vi "Launch Smart Relay Actor.vi"(8 "error in":errorcluster, 11 "SCADA in":refnum<class "EMS.lvclass">) -> (0 "error out":errorcluster, 3 "SCADA out":refnum<class "EMS.lvclass">)   [LabVIEW 2018, in "EMS Core.lvlib" / "EMS.lvclass"]
uses:
  EMS.lvclass
  C:/Users/Administrator/Desktop/LabVIEW EMS/EMS Generic Actor/EMS Generic/EMS Generic.lvclass
  C:/Program Files (x86)/National Instruments/LabVIEW 2018/vi.lib/ActorFramework/Actor/Actor.lvclass
  IED Actors/Smart Relay Actor/Smart Relay/Smart Relay.lvclass
  <vilib>/ORNL/CSEISMIC DDS/CSEISMIC DDS Base/Data Types/Controls/DeviceClass Selector.ctl
  EMS.lvclass/EMS.ctl
  <vilib>/ActorFramework/Actor/Actor.lvclass
  <vilib>/ORNL/CSEISMIC DDS/CSEISMIC DDS Base/CSEISMIC DDS.lvclass
  EMS Generic Actor/EMS Generic/EMS Generic.lvclass
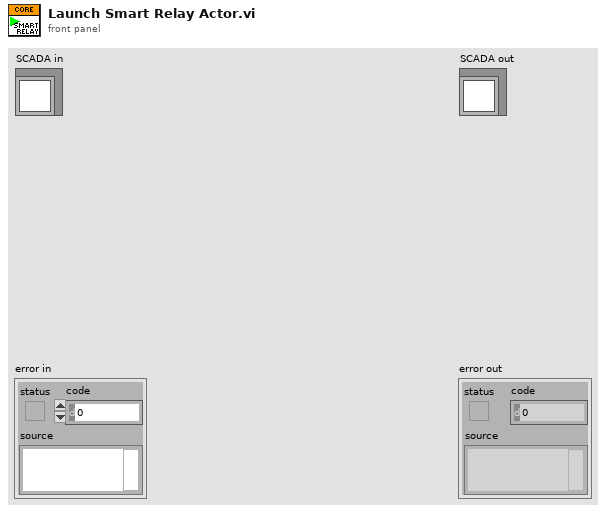
[diagram p1: front panel]
types:
  T1 = typedef "CSEISMIC DDS.lvlib/CSEISMIC DDS.lvclass/DeviceID.ctl" = string
  T2 = typedef "CSEISMIC DDS.lvlib/CSEISMIC DDS.lvclass/DeviceClass Selector.ctl" = u16
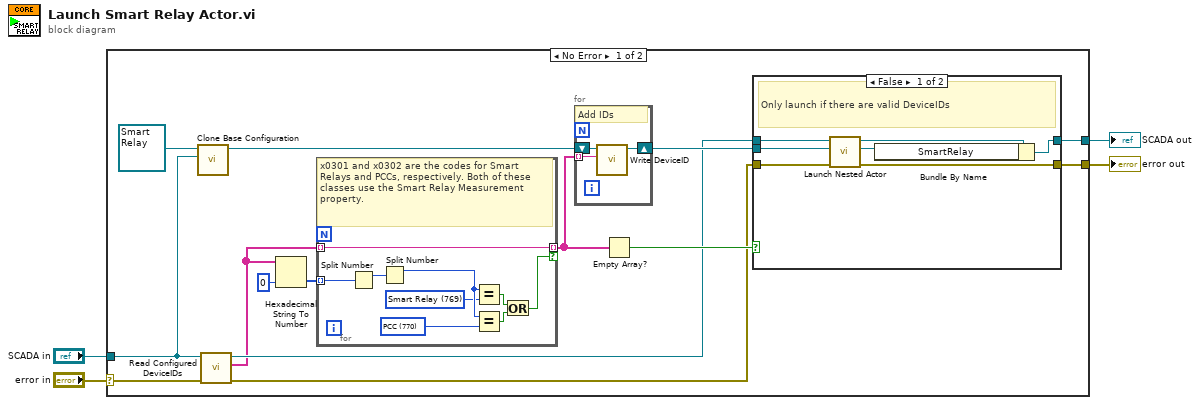
[diagram p0: block diagram]
diagram:
  n1 = case shown="No Error" "error in" {
    selector: "error in" -> [w8 w41]
    tunnel: [w17 w41] -> w3
    tunnel: [w18 w40] -> w1
    tunnel: "SCADA in" -> [w5 w40]
    frame No Error {
      n2 = call-dynamic "Clone Base Configuration.vi"("Source Object"=w5, "Target Object in"=refnum<class "Smart Relay.lvclass"> refnum ("Smart Relay Actor.lvlib:Smart Relay.lvclass")) -> ("Target Object out"=w6:refnum<class "Smart Relay.lvclass">)  [unwired: 9 in]
      n3 = call "Read Configured DeviceIDs.vi"("error in"=w8, "EMS Generic in"=w5) -> ("error out"=w12:errorcluster, "DeviceIDs"=w10:T1[], "EMS Generic out"=w13:refnum<class "EMS.lvclass">)  [unwired: 7 in]
      n4 = Hexadecimal String To Number(string=w10, default (0uL)=u64 0 ("default (0 U32)")) -> (number=w9:u64[])  [unwired: 1 in, 1 out]
      n5 = for {
        tunnel: w10 -> [w35] mode=indexing
        tunnel: [w35] -> w15 mode=indexing if=w34
        tunnel: w9 -> [w31] mode=indexing
        w32 = T2 770 items=["Invalid"=0, "IED"=256, "DER"=512, "Relay"=768, "Meter"=1024, "Load"=1280, "Energy Storage"=513, "PV"=514, "Generator"=515, "Smart Relay"=769, "PCC"=770, "Smart Meter"=1025, "PMU"=1026, "HVAC"=1281] ("DeviceClass")
        w33 = T2 769 items=["Invalid"=0, "IED"=256, "DER"=512, "Relay"=768, "Meter"=1024, "Load"=1280, "Energy Storage"=513, "PV"=514, "Generator"=515, "Smart Relay"=769, "PCC"=770, "Smart Meter"=1025, "PMU"=1026, "HVAC"=1281] ("DeviceClass")
        # "x0301 and x0302 are the codes for Smart Relays and PCCs, respectively. Both of these classes use the Smart Relay Measurement property."
        n6 = Split Number(x=w31) -> (hi(x)=w39:u32)  [unwired: 1 out]
        n7 = Split Number(x=w39) -> (hi(x)=w38:u16)  [unwired: 1 out]
        n8 = Equal?(x=w38, y=w33) -> (x = y?=w37:bool)
        n9 = Equal?(x=w38, y=w32) -> (x = y?=w36:bool)
        n10 = Or(x=w37, y=w36) -> (x .or. y?=w34:bool)
      }
      n11 = for {
        shift-right: [w29] -> w16
        shift-left: w6 -> [w30]
        tunnel: w15 -> [w28] mode=indexing
        # "Add IDs"
        n12 = call-dynamic "Write DeviceID.vi"("DeviceID"=w28, "Device DDS Communications in"=w30) -> ("Device DDS Communications out"=w29:refnum<class "Smart Relay.lvclass">)  [unwired: 9 in]
      }
      n13 = Empty Array?(array=w15) -> (empty?=w14:bool)
      n14 = case shown="False" w14 {
        tunnel: [w20 w27] -> w18
        tunnel: w12 -> [w24 w26]
        tunnel: [w23 w26] -> w17
        tunnel: w16 -> [w22 _]
        tunnel: w13 -> [w21 w27]
        frame False {
          # "Only launch if there are valid DeviceIDs"
          n15 = call <vilib>:"Launch Nested Actor.vi"("error in (no error)"=w24, "Nested Actor"=w22, "Caller Actor in"=w21) -> ("error out"=w23:errorcluster, "Nested Actor's Enqueuer"=w19:refnum<class "Message Enqueuer.lvclass">, "Caller Actor out"=w25:refnum<class "EMS.lvclass">)  [unwired: 6 in]
          n16 = Bundle By Name(cluster=w25, "SmartRelay"=w19) -> (w20:refnum<class "EMS.lvclass">)
        }
        frame True {
        }
      }
    }
    frame Error {
    }
  }
  "error out" <- w3
  "SCADA out" <- w1
